vi "ApplyLanguageToAll.vi"(8 "error in (no error)":errorcluster, 9 "Target Language":string, 10 "Dictionary":T2, 11 "VI Status":T1[](array[typedef])) -> (0 "error out":errorcluster, 3 "VI Status":T1[](array[typedef]))   [LabVIEW 2020]
uses:
  Dictionary--Cluster.ctl
  Font -- Cluster.ctl
  Phrase Dictionary Entry -- Cluster.ctl
  VI Info -- Cluster.ctl
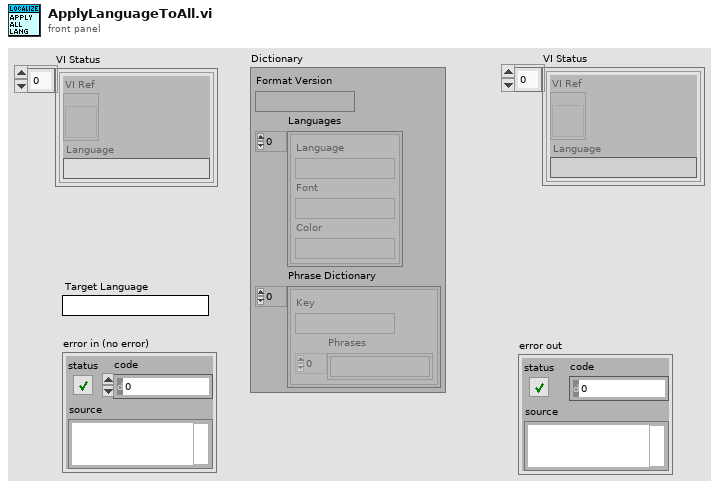
[diagram p1: front panel]
types:
  T1 = typedef "VI Info -- Cluster.ctl" = cluster{"VI Ref":refnum<vi>, "Language":string}
  T2 = typedef "Dictionary--Cluster.ctl" = cluster{"Format Version":string, "Languages":T3[], "Phrase Dictionary":T4[]}
  T3 = typedef "Font -- Cluster.ctl" = cluster{"Language":string, "Font":string, "Color":string}
  T4 = typedef "Phrase Dictionary Entry -- Cluster.ctl" = cluster{"Key":string, "Phrases":string[]}
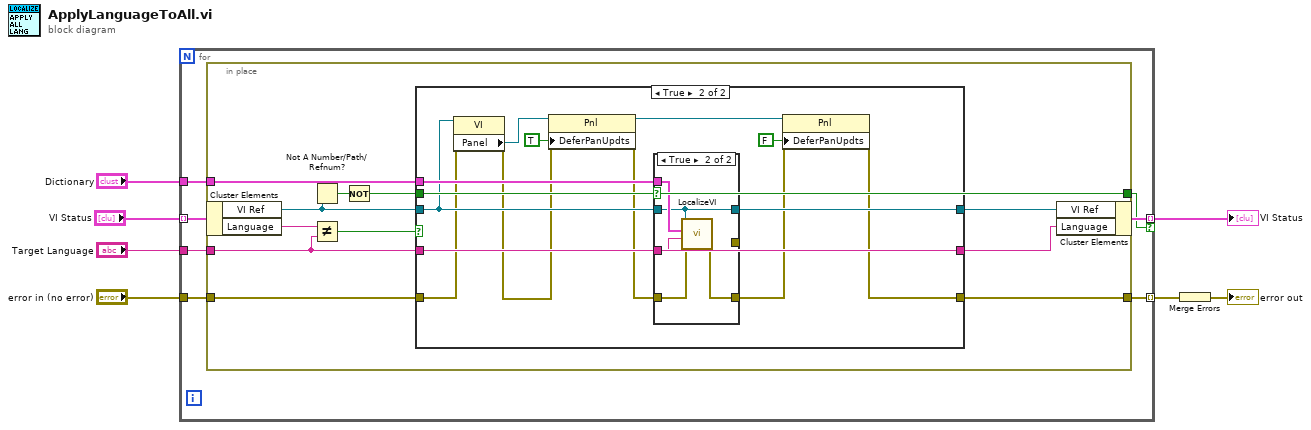
[diagram p0: block diagram]
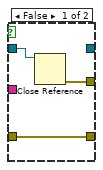
[diagram p3: hidden frame]
diagram:
  n1 = for {
    tunnel: "Dictionary" -> [w12]
    tunnel: "VI Status" -> [w10] mode=indexing
    tunnel: "Target Language" -> [w11]
    tunnel: "error in (no error)" -> [w14]
    tunnel: [w13] -> w4 mode=indexing
    tunnel: [w9] -> w1 mode=indexing if=w8
    n2 = in-place {
      in-place-border: w14 -> [w25]
      in-place-border: [w24] -> w13
      in-place-border: w12 -> [w23]
      in-place-border: w11 -> [w21]
      in-place-border: [w15] -> w8
      n3 = in-place-cluster #1(w10) -> ("VI Ref"=w19:refnum<vi>, "Language"=w18:string)
      n4 = Not A Number/Path/Refnum?(number/path/refnum=w19) -> (NaN/Path/Refnum?=w22:bool)
      n5 = Not Equal?(x=w18, y=w21) -> (x != y?=w20:bool)
      n6 = Not(x=w22) -> (.not. x?=w15:bool)
      n7 = case shown="True" w20 {
        tunnel: w25 -> [w28 w35]
        tunnel: [w28 w29] -> w24
        tunnel: w23 -> [_ w42]
        tunnel: w15 -> [_ w41]
        tunnel: w19 -> [w27 w36]
        tunnel: w21 -> [w26 w40]
        tunnel: [w27 w39] -> w17
        tunnel: [w26 w40] -> w16
        frame False {
        }
        frame True {
          n8 = property class="VI"(reference=w36, error in=w35) -> (error out=w34:errorcluster, "Panel"=w38:refnum<vi>)  [unwired: 1 out]
          n9 = property class="Pnl"(reference=w38, error in=w34, "DeferPanUpdts"=TRUE ("Defer Panel Updates")) -> (reference out=w32:refnum<vi>, error out=w33:errorcluster)
          n10 = case shown="True" w41 {
            tunnel: w33 -> [w45 w50]
            tunnel: [w45 w49] -> w30
            tunnel: w42 -> [_ w48]
            tunnel: w40 -> [_ w47]
            tunnel: w36 -> [w44 w46]
            tunnel: [w43 _] -> _
            tunnel: [_ w46] -> w39
            frame False {
              n11 = Close Reference(reference=w44) -> (error out=w43:errorcluster)  [unwired: 1 in]
            }
            frame True {
              n12 = call "LocalizeVI.vi"("error in (no error)"=w50, "Target Language"=w47, "Dictionary"=w48, "VI in"=w46) -> ("error out"=w49:errorcluster)  [unwired: 7 in]
            }
          }
          n13 = property class="Pnl"(reference=w32, error in=w30, "DeferPanUpdts"=FALSE ("Defer Panel Updates")) -> (error out=w29:errorcluster)  [unwired: 1 out]
        }
      }
      n14 = in-place-cluster #1("VI Ref"=w17, "Language"=w16) -> (w9:T1)
    }
  }
  "VI Status" <- w1
  n15 = Merge Errors(w4) -> (→"error out":errorcluster)
